vi "Create Messaging Structure.vi"(8 "error in (no error)":errorcluster) -> (0 "error out":errorcluster, 3 "Events":T1)   [LabVIEW 2018, in "Launcher.lvlib"]
uses:
  Launcher.lvlib
  Event Message Cluster.ctl
  Module/User Event Message Cluster.ctl
  Module/User Event Message Enum.ctl
  Error Handler/User Event Message Cluster.ctl
  Error Handler/User Event Message Enum.ctl
  Error Handler/Event Ref FGV Command Enum.ctl
  Shutdown Event FGV Command.ctl
  Error Handler/Error Handler.lvlib
  Module/Template Module.lvlib
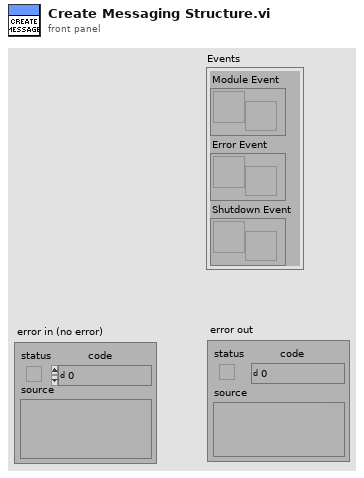
[diagram p1: front panel]
types:
  T1 = typedef "Launcher.lvlib/Event Message Cluster.ctl" = cluster{"Module Event":refnum<user-event>, "Error Event":refnum<user-event>, "Shutdown Event":refnum<user-event>}
  T2 = typedef "Launcher.lvlib/Shutdown Event FGV Command.ctl" = enum16{"Create Event", "Get Event Ref", "Release Event"}
  T3 = typedef "Error Handler.lvlib/Event Ref FGV Command Enum.ctl" = enum16{"Create Event", "Get Event Ref", "Release Event"}
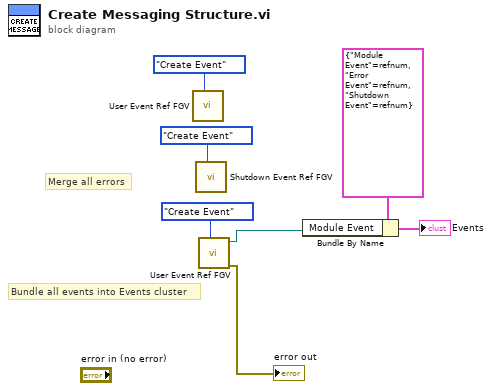
[diagram p0: block diagram]
diagram:
  # "Merge all errors"
  # "Bundle all events into Events cluster"
  n1 = call "User Event Ref FGV.vi"("Command"=Event_Ref_FGV_Command_Enum."Create Event") -> ()  [unwired: 9 in, 2 out]
  n2 = call "Shutdown Event Ref FGV.vi"("Command"=Shutdown_Event_FGV_Command."Create Event") -> ()  [unwired: 9 in, 2 out]
  n3 = call "User Event Ref FGV.vi"("Command"=Event_Ref_FGV_Command_Enum."Create Event") -> ("error out"=→"error out":errorcluster, "User Event"=w5:refnum<user-event>)  [unwired: 9 in]
  n4 = Bundle By Name(cluster=T1 {"Module Event"=refnum, "Error Event"=refnum, "Shutdown Event"=refnum} ("Cluster"), "Module Event"=w5) -> (→"Events":T1)
